vi "Write Camara.vi"(8 "error in (no error)":errorcluster, 10 "Camara":string, 11 "Webcam in":refnum<class "Webcam.lvclass">) -> (0 "error out":errorcluster, 3 "Webcam out":refnum<class "Webcam.lvclass">)   [LabVIEW 2020, in "Webcam.lvclass"]
uses:
  Webcam.lvclass
  Webcam.lvclass/Webcam.ctl
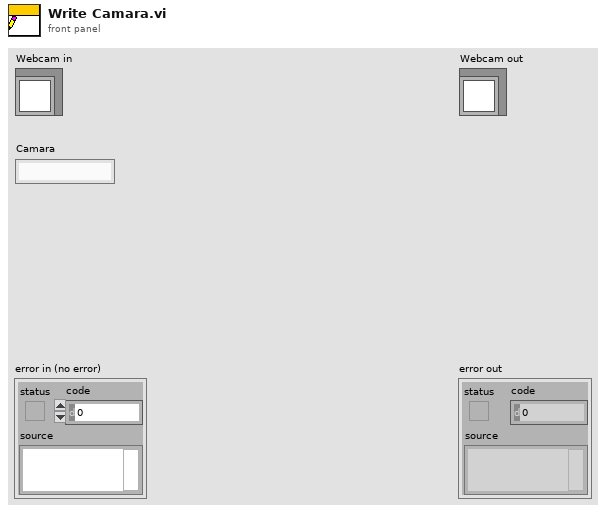
[diagram p1: front panel]
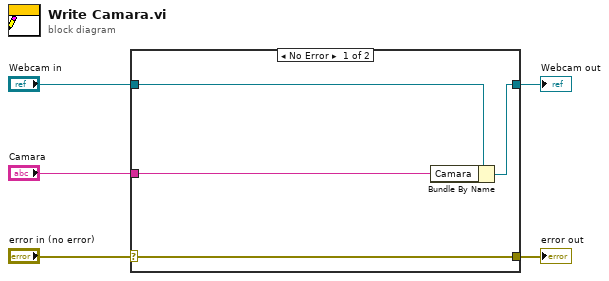
[diagram p0: block diagram]
diagram:
  n1 = case shown="No Error" "error in (no error)" {
    selector: "error in (no error)" -> [w9 w10]
    tunnel: [w9 w10] -> w4
    tunnel: [w7 w11] -> w2
    tunnel: "Webcam in" -> [w8 w11]
    tunnel: "Camara" -> [w6 _]
    frame No Error {
      n2 = Bundle By Name(cluster=w8, "Camara"=w6) -> (w7:refnum<class "Webcam.lvclass">)
    }
    frame Error {
    }
  }
  "error out" <- w4
  "Webcam out" <- w2
